vi "Scale DAQ Data.vi"(0 "Data Read":sgl[][](array[numeric]), 5 "Coefficients":T2, 7 "System Type":T1, 12 "Sensor (scaling)":T3(array[cluster]), 13 "mA Shunt":bool) -> (4 "Scaled Data":sgl[][](array[numeric]))   [LabVIEW 2023]
uses:
  Type Defs and Controls/Coeffs Cluster Type Def.ctl
  Type Defs and Controls/System Type.ctl
  <vilib>/Analysis/NI_AALBase.lvlib
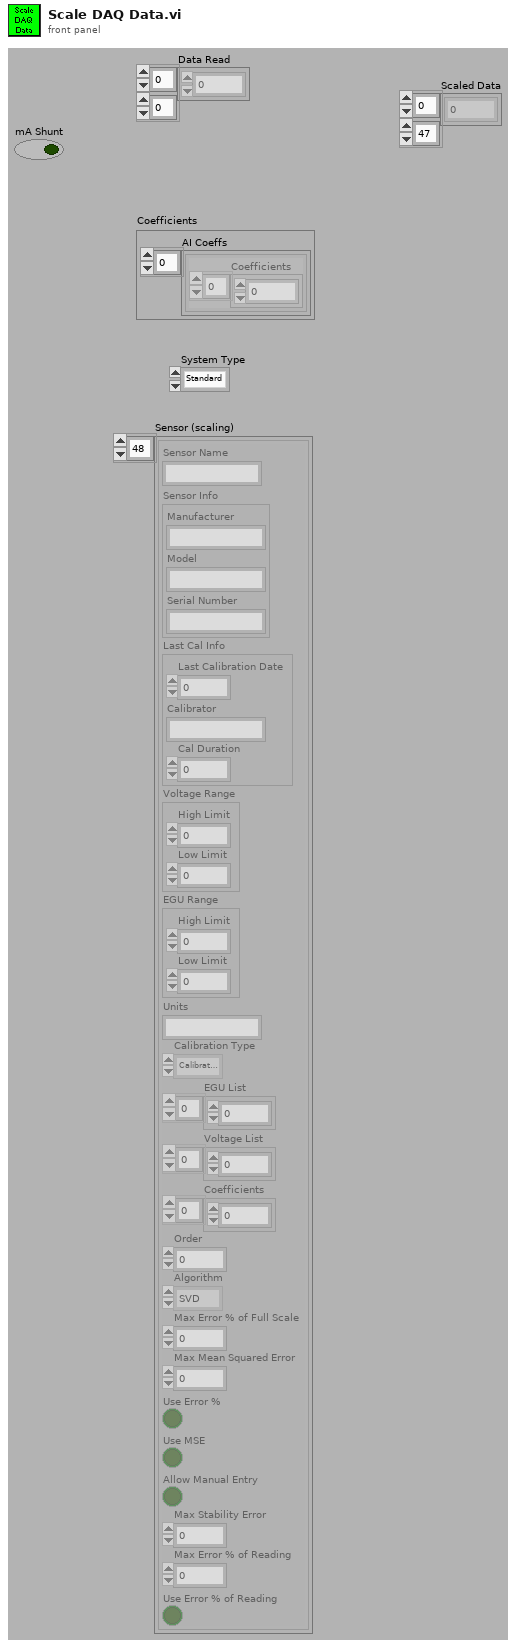
[diagram p1: front panel]
types:
  T1 = typedef "System Type.ctl" = enum16{"Standard", "Deformation", "Standard 8TC"}
  T2 = typedef "Coeffs Cluster Type Def.ctl" = cluster{"AI Coeffs":cluster{"Coefficients":dbl[]}[]}
  T3 = cluster{"Sensor Name":string, "Sensor Info":cluster{"Manufacturer":string, "Model":string, "Serial Number":string}, "Last Cal Info":cluster{"Last Calibration Date":dbl, "Calibrator":string, "Cal Duration":i32}, "Voltage Range":cluster{"High Limit":dbl, "Low Limit":dbl}, "EGU Range":cluster{"High Limit":dbl, "Low Limit":dbl}, "Units":string, "Calibration Type":enum16{"Calibrate Analog", "Compare Analog Calibration"}, "EGU List":dbl[], "Voltage List":dbl[], "Coefficients":dbl[], "Order":i32, "Algorithm":enum32{"SVD", "Givens", "Givens2", "Householder", "LU Decomposition", "Cholesky"}, "Max Error % of Full Scale":dbl, "Max Mean Squared Error":dbl, "Use Error %":bool, "Use MSE":bool, "Allow Manual Entry":bool, "Max Stability Error":dbl, "Max Error % of Reading":dbl, "Use Error % of Reading":bool}[]
  T4 = cluster{"Sensor Name":string, "Sensor Info":cluster{"Manufacturer":string, "Model":string, "Serial Number":string}, "Last Cal Info":cluster{"Last Calibration Date":dbl, "Calibrator":string, "Cal Duration":i32}, "Voltage Range":cluster{"High Limit":dbl, "Low Limit":dbl}, "EGU Range":cluster{"High Limit":dbl, "Low Limit":dbl}, "Units":string, "Calibration Type":enum16{"Calibrate Analog", "Compare Analog Calibration"}, "EGU List":dbl[], "Voltage List":dbl[], "Coefficients":dbl[], "Order":i32, "Algorithm":enum32{"SVD", "Givens", "Givens2", "Householder", "LU Decomposition", "Cholesky"}, "Max Error % of Full Scale":dbl, "Max Mean Squared Error":dbl, "Use Error %":bool, "Use MSE":bool, "Allow Manual Entry":bool, "Max Stability Error":dbl, "Max Error % of Reading":dbl, "Use Error % of Reading":bool}
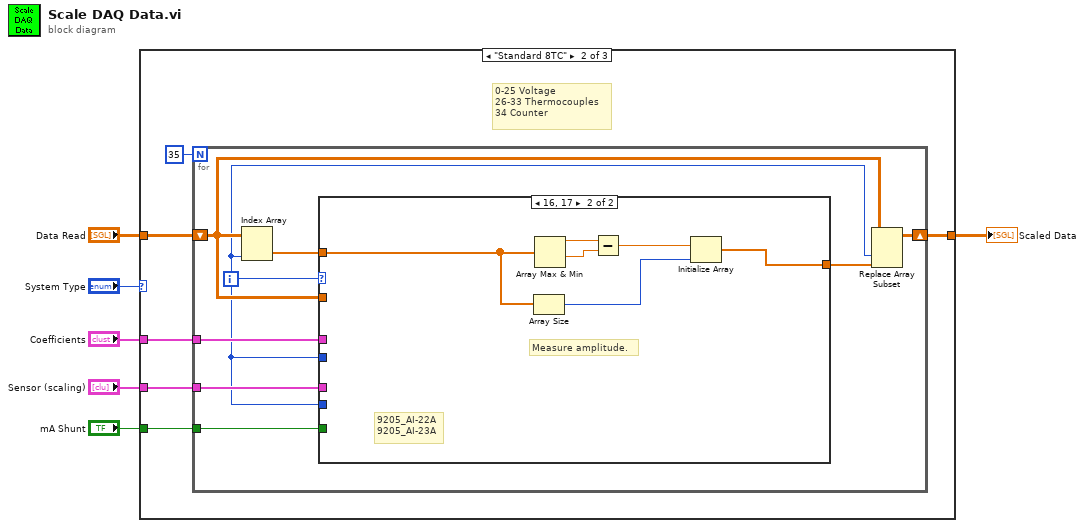
[diagram p0: block diagram]
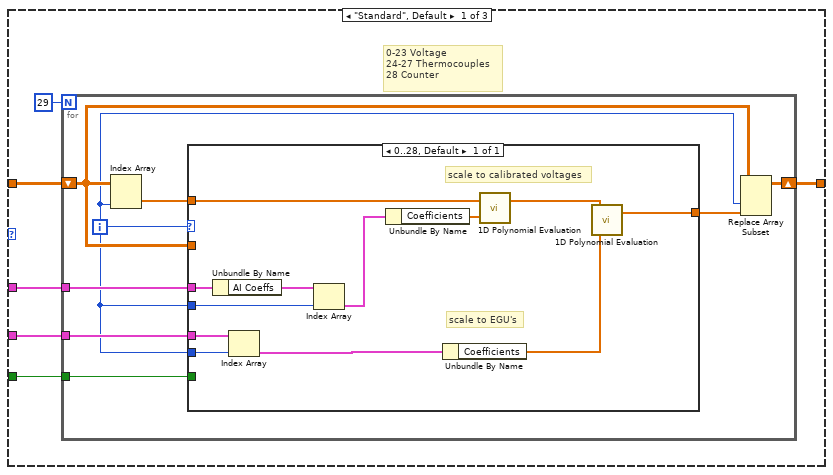
[diagram p2: hidden frame]
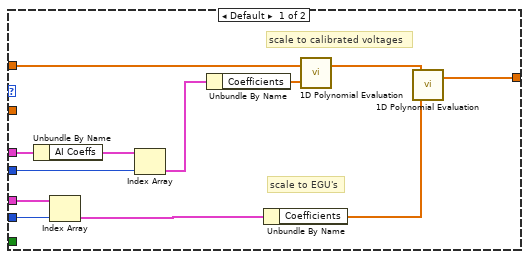
[diagram p3: hidden frame]
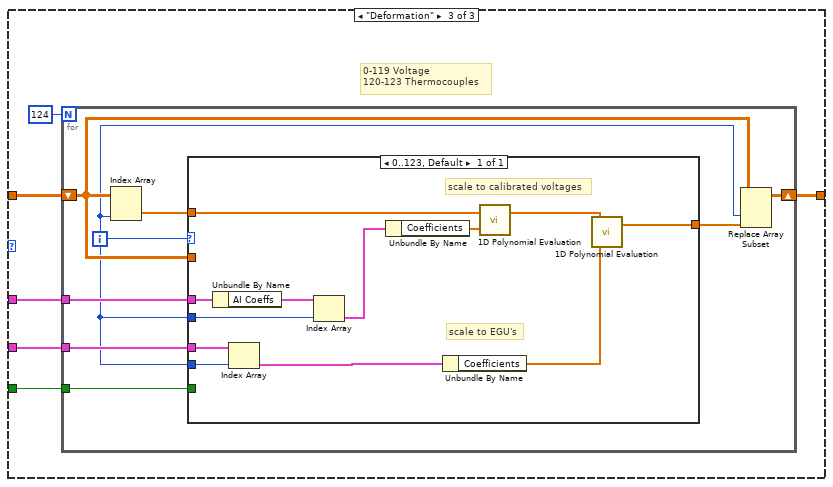
[diagram p4: hidden frame]
diagram:
  n1 = case shown="\"Standard 8TC\"" "System Type" {
    tunnel: "Sensor (scaling)" -> [w12 w38 w70]
    tunnel: "Coefficients" -> [w11 w37 w69]
    tunnel: "Data Read" -> [w10 w36 w68]
    tunnel: [w8 w34 w66] -> w3
    tunnel: "mA Shunt" -> [w7 w33 w65]
    frame "Standard", Default {
      # "0-23 Voltage\n24-27 Thermocouples\n28 Counter"
      n2 = for {
        N: 29 -> [_]
        tunnel: w11 -> [w16]
        shift-right: [w19] -> w8
        shift-left: w10 -> [w17]
        tunnel: w12 -> [w14]
        tunnel: w7 -> [w15]
        i -> [w13]
        n3 = Index Array(array=w17, index (col)=w13) -> (element=w20:sgl[])  [unwired: 1 in]
        n4 = case shown="0..28, Default" w13 {
          tunnel: w20 -> [w32]
          tunnel: [w28] -> w18
          tunnel: w17 -> [_]
          tunnel: w16 -> [w27]
          tunnel: w13 -> [w25]
          tunnel: w15 -> [_]
          tunnel: w14 -> [w23]
          tunnel: w13 -> [w21]
          frame 0..28, Default {
            # "scale to calibrated voltages"
            # "scale to EGU's"
            n5 = Unbundle By Name(w27) -> ("AI Coeffs"=w26:cluster{"Coefficients":dbl[]}[])
            n6 = Index Array(array=w23, index=w21) -> (element=w22:T4)
            n7 = Index Array(array=w26, index=w25) -> (element=w24:cluster{"Coefficients":dbl[]})
            n8 = Unbundle By Name(w24) -> ("Coefficients"=w31:dbl[])
            n9 = Unbundle By Name(w22) -> ("Coefficients"=w29:dbl[])
            n10 = call <vilib>:"1D Polynomial Evaluation.vi"("Coefficients: a"=w31, "X"=w32) -> ("Y"=w30:dbl[])  [unwired: 1 out]
            n11 = call <vilib>:"1D Polynomial Evaluation.vi"("Coefficients: a"=w29, "X"=w30) -> ("Y"=w28:dbl[])  [unwired: 1 out]
          }
        }
        n12 = Replace Array Subset(array=w17, new element=w18, index (col)=w13) -> (w19:sgl[][])  [unwired: 1 in]
      }
    }
    frame "Standard 8TC" {
      # "0-25 Voltage\n26-33 Thermocouples\n34 Counter"
      n13 = for {
        N: 35 -> [_]
        tunnel: w37 -> [w42]
        shift-right: [w45] -> w34
        shift-left: w36 -> [w43]
        tunnel: w38 -> [w40]
        tunnel: w33 -> [w41]
        i -> [w39]
        n14 = Index Array(array=w43, index (col)=w39) -> (element=w46:sgl[])  [unwired: 1 in]
        n15 = case shown="16, 17" w39 {
          tunnel: w46 -> [w58 w61]
          tunnel: [w54 w59] -> w44
          tunnel: w43 -> [_ _]
          tunnel: w42 -> [w53 _]
          tunnel: w39 -> [w51 _]
          tunnel: w41 -> [_ _]
          tunnel: w40 -> [w49 _]
          tunnel: w39 -> [w47 _]
          frame Default {
            # "scale to calibrated voltages"
            # "scale to EGU's"
            n16 = Unbundle By Name(w53) -> ("AI Coeffs"=w52:cluster{"Coefficients":dbl[]}[])
            n17 = Index Array(array=w49, index=w47) -> (element=w48:T4)
            n18 = Index Array(array=w52, index=w51) -> (element=w50:cluster{"Coefficients":dbl[]})
            n19 = Unbundle By Name(w50) -> ("Coefficients"=w57:dbl[])
            n20 = Unbundle By Name(w48) -> ("Coefficients"=w55:dbl[])
            n21 = call <vilib>:"1D Polynomial Evaluation.vi"("Coefficients: a"=w57, "X"=w58) -> ("Y"=w56:dbl[])  [unwired: 1 out]
            n22 = call <vilib>:"1D Polynomial Evaluation.vi"("Coefficients: a"=w55, "X"=w56) -> ("Y"=w54:dbl[])  [unwired: 1 out]
          }
          frame 16, 17 {
            # "Measure amplitude."
            # "9205_AI-22A\n9205_AI-23A"
            n23 = Array Size(array=w61) -> (size(s)=w60:i32)
            n24 = Array Max & Min(array=w61) -> (max value=w64:sgl, min value=w63:sgl)  [unwired: 2 out]
            n25 = Subtract(x=w64, y=w63) -> (x-y=w62:sgl)
            n26 = Initialize Array(w62, w60) -> (w59:sgl[])
          }
        }
        n27 = Replace Array Subset(array=w43, new element=w44, index (col)=w39) -> (w45:sgl[][])  [unwired: 1 in]
      }
    }
    frame "Deformation" {
      # "0-119 Voltage\n120-123 Thermocouples"
      n28 = for {
        N: 124 -> [_]
        tunnel: w69 -> [w74]
        shift-right: [w77] -> w66
        shift-left: w68 -> [w75]
        tunnel: w70 -> [w72]
        tunnel: w65 -> [w73]
        i -> [w71]
        n29 = Index Array(array=w75, index (col)=w71) -> (element=w78:sgl[])  [unwired: 1 in]
        n30 = case shown="0..123, Default" w71 {
          tunnel: w78 -> [w90]
          tunnel: [w86] -> w76
          tunnel: w75 -> [_]
          tunnel: w74 -> [w85]
          tunnel: w71 -> [w83]
          tunnel: w73 -> [_]
          tunnel: w72 -> [w81]
          tunnel: w71 -> [w79]
          frame 0..123, Default {
            # "scale to calibrated voltages"
            # "scale to EGU's"
            n31 = Unbundle By Name(w85) -> ("AI Coeffs"=w84:cluster{"Coefficients":dbl[]}[])
            n32 = Index Array(array=w81, index=w79) -> (element=w80:T4)
            n33 = Index Array(array=w84, index=w83) -> (element=w82:cluster{"Coefficients":dbl[]})
            n34 = Unbundle By Name(w82) -> ("Coefficients"=w89:dbl[])
            n35 = Unbundle By Name(w80) -> ("Coefficients"=w87:dbl[])
            n36 = call <vilib>:"1D Polynomial Evaluation.vi"("Coefficients: a"=w89, "X"=w90) -> ("Y"=w88:dbl[])  [unwired: 1 out]
            n37 = call <vilib>:"1D Polynomial Evaluation.vi"("Coefficients: a"=w87, "X"=w88) -> ("Y"=w86:dbl[])  [unwired: 1 out]
          }
        }
        n38 = Replace Array Subset(array=w75, new element=w76, index (col)=w71) -> (w77:sgl[][])  [unwired: 1 in]
      }
    }
  }
  "Scaled Data" <- w3
